vi "Process Regular Signal.vi"(9 "Values Received":dbl[](array[numeric]), 10 "Incoming Values In":T1, 11 "Frame Settings In":T2 {"Protection Configurations"."CRC Channels"."Data Type" items=["Signed", "Unsigned", "IEEE Float"]}) -> (2 "Incoming Values Out":T1, 3 "Frame Settings Out":T2 {"Protection Configurations"."CRC Channels"."Data Type" items=["Signed", "Unsigned", "IEEE Float"]})   [LabVIEW 2019, in "Protection and Counter Addon Engine.lvlib"]
uses:
  Protection and Counter Addon Engine.lvlib
  SubModules/Frame-Protection-Support/Source/Engine/Types/RT Frame Settings.ctl
  SubModules/Frame-Protection-Support/Source/Shared/Types/Exported Frame Type.ctl
  SubModules/Frame-Protection-Support/Source/Engine/Types/RT Protection Configuration.ctl
  SubModules/Frame-Protection-Support/Source/Shared/Types/Protection Type.ctl
  SubModules/Frame-Protection-Support/Source/Shared/Types/XNET Signal Configuration.ctl
  SubModules/Frame-Protection-Support/Source/Shared/Types/Exported Counter Settings.ctl
  SubModules/Frame-Protection-Support/Source/Shared/Types/Exported Event Trigger Type.ctl
  Types/Incoming Values.ctl
  SubModules/Frame-Protection-Support/Source/Shared/Protection and Counter Support Shared.lvlib
  SubModules/Frame-Protection-Support/Source/Engine/Protection and Counter Support Engine.lvlib
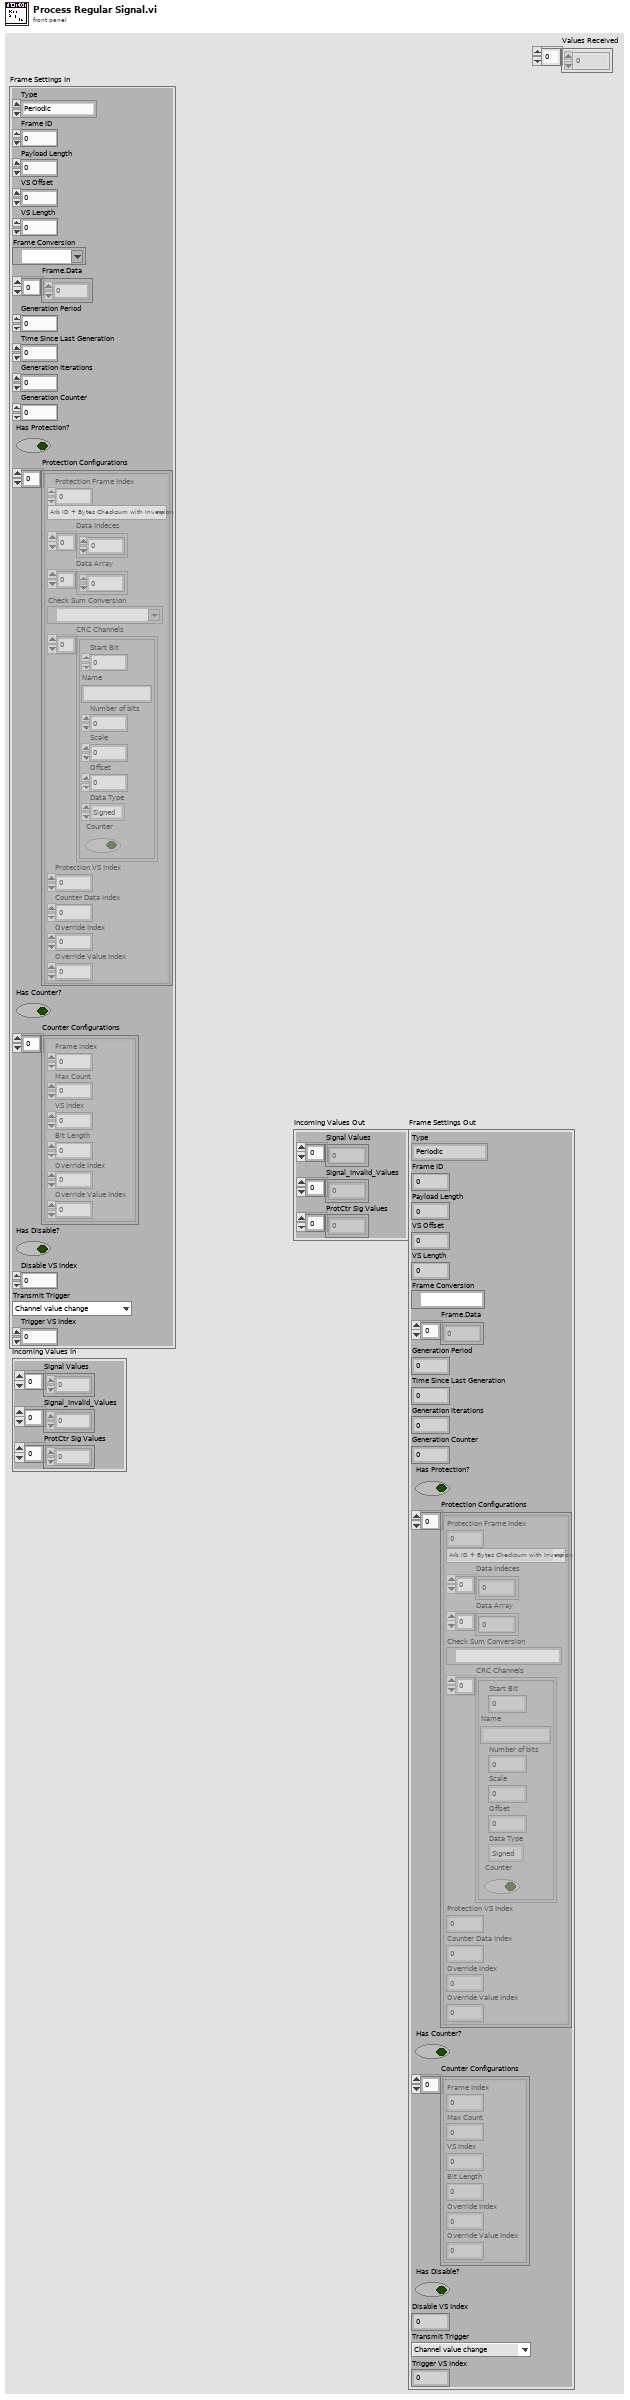
[diagram p1: front panel]
types:
  T1 = typedef "Protection and Counter Addon Engine.lvlib/Incoming Values.ctl" = cluster{"Signal Values":dbl[], "Signal_Invalid_Values":dbl[], "ProtCtr Sig Values":dbl[]}
  T2 = typedef "Protection and Counter Support Engine.lvlib/RT Frame Settings.ctl" = cluster{"Type":T3, "Frame ID":u32, "Payload Length":u32, "VS Offset":i32, "VS Length":i32, "Frame Conversion":refnum<k21>, "Frame.Data":dbl[], "Generation Period":u32, "Time Since Last Generation":u32, "Generation Iterations":u32, "Generation Counter":u32, "Has Protection?":bool, "Protection Configurations":T4[], "Has Counter?":bool, "Counter Configurations":T7[], "Has Disable?":bool, "Disable VS Index":i32, "Transmit Trigger":T8, "Trigger VS Index":i32}
  T3 = typedef "Protection and Counter Support Shared.lvlib/Exported Frame Type.ctl" = enum16{"Periodic", "Event", "Periodic/Event"}
  T4 = typedef "Protection and Counter Support Engine.lvlib/RT Protection Configuration.ctl" = cluster{"Protection Frame Index":i32, "Protection Type":T5, "Data Indeces":i32[], "Data Array":dbl[], "Check Sum Conversion":refnum<k21>, "CRC Channels":T6[], "Protection VS Index":i32, "Counter Data Index":i32, "Override Index":i32, "Override Value Index":i32}
  T5 = typedef "Protection and Counter Support Shared.lvlib/Protection Type.ctl" = enum16{"Arb ID + Bytes Checksum with Inversion", "Arb ID + Bytes CRC with Inversion", "Reversed Raw Signal Checksum with Inversion", "Concatenated Two's Compliment"}
  T6 = typedef "Protection and Counter Support Shared.lvlib/XNET Signal Configuration.ctl" = cluster{"Start Bit":i32, "Name":string, "Number of bits":i32, "Scale":dbl, "Offset":dbl, "Data Type":u32, "Counter":bool}
  T7 = typedef "Protection and Counter Support Shared.lvlib/Exported Counter Settings.ctl" = cluster{"Frame Index":i32, "Max Count":dbl, "VS Index":i32, "Bit Length":i64, "Override Index":i32, "Override Value Index":i32}
  T8 = typedef "Protection and Counter Support Shared.lvlib/Exported Event Trigger Type.ctl" = enum16{"Channel value change", "Trigger channel (not zero)", "Channel value change or trigger channel (not zero)", "Trigger channel (any value change)", "Channel value change or trigger channel (any value change)"}
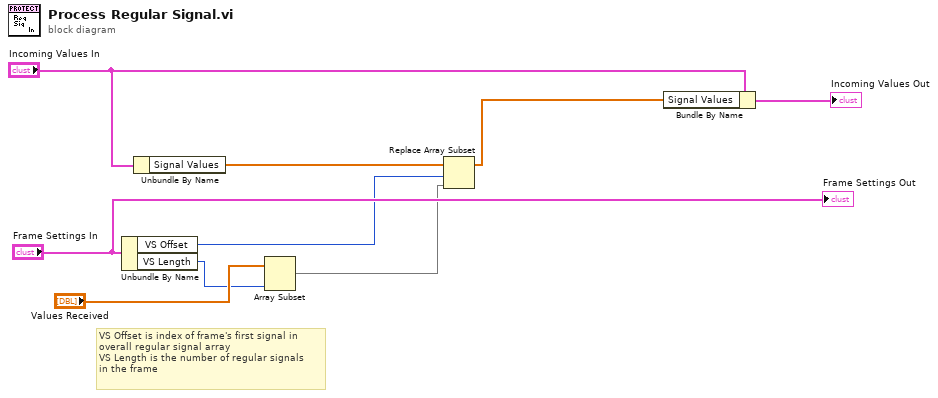
[diagram p0: block diagram]
diagram:
  # "VS Offset is index of frame's first signal in\noverall regular signal array\nVS Length is the number of regular signals \nin the frame"
  n1 = Unbundle By Name("Frame Settings In") -> ("VS Offset"=w8:i32, "VS Length"=w6:i32)
  n2 = Unbundle By Name("Incoming Values In") -> ("Signal Values"=w2:dbl[])
  n3 = Array Subset(array="Values Received", length=w6) -> (w5:dbl[])  [unwired: 1 in]
  n4 = Replace Array Subset(array=w2, new element=w5, index=w8) -> (w1:dbl[])
  n5 = Bundle By Name(cluster="Incoming Values In", "Signal Values"=w1) -> (→"Incoming Values Out":T1)
  "Frame Settings Out" <- "Frame Settings In"
